vi "Get Sinks from Array.vi"(8 "error in (no error)":errorcluster, 11 "Registry in":refnum<class "Registry.lvclass">) -> (0 "error out":errorcluster, 2 "Sinks":refnum<class "Sink.lvclass">[](array[class]), 3 "Registry out":refnum<class "Registry.lvclass">)   [LabVIEW 2025, in "LV Logging.lvlib" / "Registry.lvclass"]
uses:
  Registry.lvclass
  Sink/Sink.lvclass
  Registry.lvclass/Registry.ctl
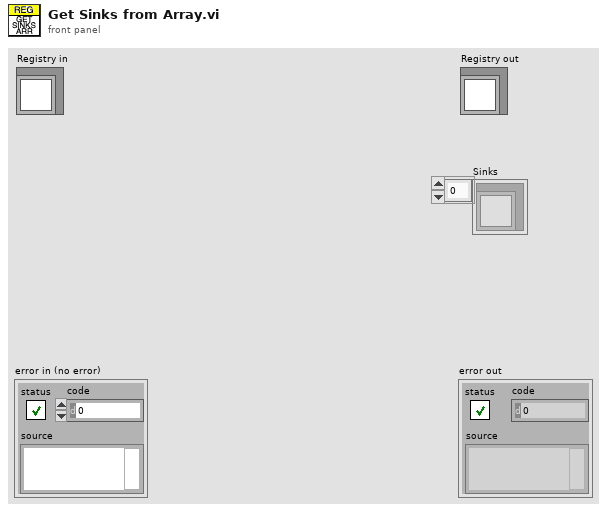
[diagram p1: front panel]
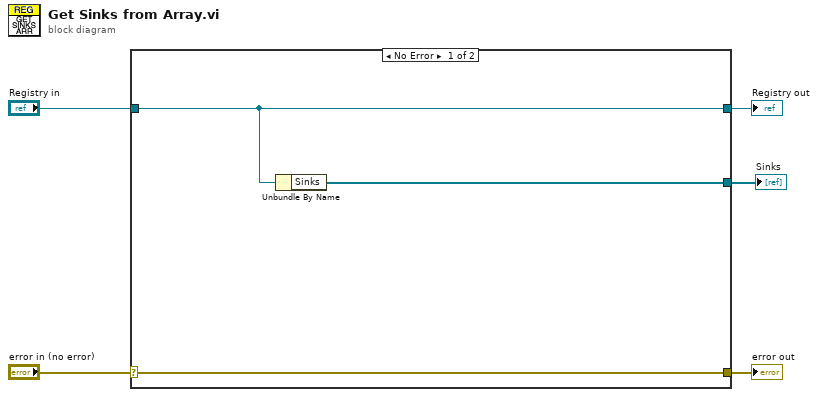
[diagram p0: block diagram]
diagram:
  n1 = case shown="No Error" "error in (no error)" {
    selector: "error in (no error)" -> [w8 w10]
    tunnel: [w8 w10] -> w4
    tunnel: [w7 w9] -> w2
    tunnel: "Registry in" -> [w7 w9]
    tunnel: [w6 _] -> w1
    frame No Error {
      n2 = Unbundle By Name(w7) -> ("Sinks"=w6:refnum<class "Sink.lvclass">[])
    }
    frame Error {
    }
  }
  "error out" <- w4
  "Registry out" <- w2
  "Sinks" <- w1
